vi "I32 to U64 2D-Array.vi"(1 "I32 Array":i32[][](array[numeric])) -> (0 "Array of U64 cast as DBLs":dbl[][](array[numeric]))   [LabVIEW 2017]
panel:
  # "LVHDF5 Toolkit\nCopyright (c) 2005-2013 by Jason D. Sommerville\nCopyright (c) 2014 by UPVI, LLC.\n\nThis use and distribution of this file is governed by the terms found in \nLICENSE.txt distributed with this toolkit and installed at\n <user.lib>\\_lvhdf5\\LICENSE.txt"
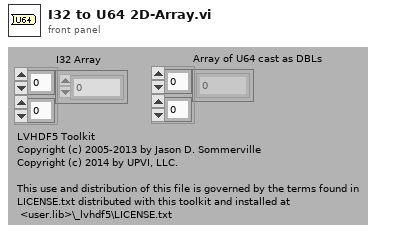
[diagram p1: front panel]
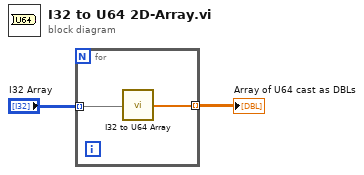
[diagram p0: block diagram]
diagram:
  n1 = for {
    tunnel: "I32 Array" -> [w4] mode=indexing
    tunnel: [w3] -> w1 mode=indexing
    n2 = call <vilib>:"I32 to U64 Array.vi"("I32 Array"=w4) -> ("Array of U64 cast as DBLs"=w3:dbl[])
  }
  "Array of U64 cast as DBLs" <- w1
